vi "Register gRPC Methods.vi"(8 "error in (no error)":errorcluster, 11 "Template Server in":refnum<class "TestService.lvclass">) -> (0 "error out":errorcluster, 3 "Template Server out":refnum<class "TestService.lvclass">)   [LabVIEW 2021, in "test_service_server.lvlib" / "TestService.lvclass"]
uses:
  TestService.lvclass
  typeDefs/Server Internal UEs.ctl
  typeDefs/Server Internal Message.ctl
  typeDefs/Server gRPC UEs.ctl
  <vilib>/gRPC/LabVIEW gRPC Library/Server API/typeDefs/gRPCId Cluster.ctl
  <vilib>/gRPC/LabVIEW gRPC Library/Shared/grpcId.ctl
  TestService.lvclass/TestService.ctl
  <vilib>/gRPC/LabVIEW gRPC Library/grpc-lvsupport-release.lvlib
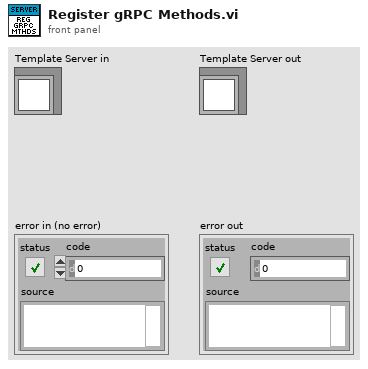
[diagram p1: front panel]
types:
  T1 = typedef "test_service_server.lvlib/TestService.lvclass/Server gRPC UEs.ctl" = cluster{"TestService Method1 gRPC UE":refnum<user-event>, "TestService Method2 gRPC UE":refnum<user-event>, "TestService Method3 gRPC UE":refnum<user-event>, "TestService Method4 gRPC UE":refnum<user-event>}
  T2 = typedef "test_service_server.lvlib/TestService.lvclass/Server Internal UEs.ctl" = cluster{"TestService Method1 Internal UE":refnum<user-event>, "TestService Method2 Internal UE":refnum<user-event>, "TestService Method3 Internal UE":refnum<user-event>, "TestService Method4 Internal UE":refnum<user-event>}
  T3 = typedef "grpc-lvsupport-release.lvlib/grpcId.ctl" = u64
  T4 = typedef "test_service_server.lvlib/TestService.lvclass/Server Internal Message UE.ctl" = refnum<user-event>
  T5 = typedef "grpc-lvsupport-release.lvlib/gRPCId Cluster UE.ctl" = refnum<user-event>
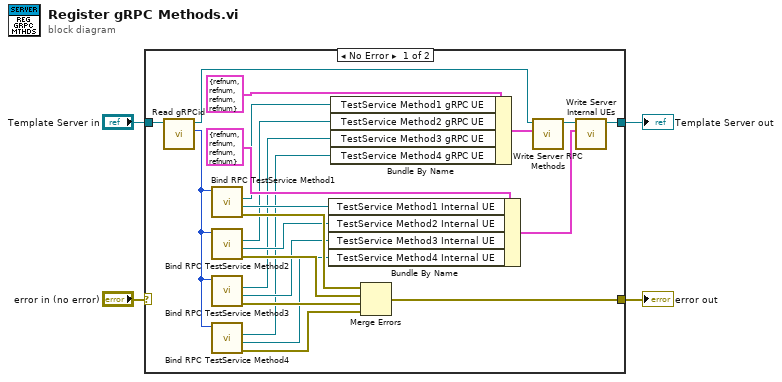
[diagram p0: block diagram]
diagram:
  n1 = case shown="No Error" "error in (no error)" {
    selector: "error in (no error)" -> [_ w27]
    tunnel: "Template Server in" -> [w18 w28]
    tunnel: [w26 w27] -> w3
    tunnel: [w25 w28] -> w2
    frame No Error {
      n2 = call-dynamic "Read gRPCid.vi"("iService in"=w18) -> ("gRPCid"=w17:T3, "iService out"=w19:refnum<class "TestService.lvclass">)  [unwired: 8 in, 1 out]
      n3 = call "Bind RPC TestService Method1.vi"("gRPCid server in"=w17) -> ("error out"=w16:errorcluster, "TestService Method1 Internal UE"=w14:T4, "TestService Method1 gRPC UE"=w15:T5)  [unwired: 7 in, 1 out]
      n4 = call "Bind RPC TestService Method2.vi"("gRPCid server in"=w17) -> ("error out"=w13:errorcluster, "TestService Method2 Internal UE"=w11:T4, "TestService Method2 gRPC UE"=w12:T5)  [unwired: 7 in, 1 out]
      n5 = call "Bind RPC TestService Method3.vi"("gRPCid server in"=w17) -> ("error out"=w10:errorcluster, "TestService Method3 Internal UE"=w8:T4, "TestService Method3 gRPC UE"=w9:T5)  [unwired: 7 in, 1 out]
      n6 = call "Bind RPC TestService Method4.vi"("gRPCid server in"=w17) -> ("error out"=w7:errorcluster, "TestService Method4 Internal UE"=w5:T4, "TestService Method4 gRPC UE"=w6:T5)  [unwired: 7 in, 1 out]
      n7 = Bundle By Name ("Bundle Internal UEs")(cluster=T2 {"TestService Method1 Internal UE"=refnum, "TestService Method2 Internal UE"=refnum, "TestService Method3 Internal UE"=refnum, "TestService Method4 Internal UE"=refnum} ("Server Internal UEs"), "TestService Method1 Internal UE"=w14, "TestService Method2 Internal UE"=w11, "TestService Method3 Internal UE"=w8, "TestService Method4 Internal UE"=w5) -> (w24:T2)
      n8 = Bundle By Name ("Bundle gRPC UEs")(cluster=T1 {"TestService Method1 gRPC UE"=refnum, "TestService Method2 gRPC UE"=refnum, "TestService Method3 gRPC UE"=refnum, "TestService Method4 gRPC UE"=refnum} ("gRPC Server Method Events"), "TestService Method1 gRPC UE"=w15, "TestService Method2 gRPC UE"=w12, "TestService Method3 gRPC UE"=w9, "TestService Method4 gRPC UE"=w6) -> (w21:T1)
      n9 = Merge Errors(w16, w13, w10, w7) -> (w26:errorcluster)
      n10 = call "Write Server RPC Methods.vi"("Server RPC Methods"=w21, "SignalGeneratorService in"=w19) -> ("SignalGeneratorService out"=w22:refnum<class "TestService.lvclass">)  [unwired: 8 in, 1 out]
      n11 = call "Write Server Internal UEs.vi"("Server Internal UEs"=w24, "SignalGeneratorService in"=w22) -> ("SignalGeneratorService out"=w25:refnum<class "TestService.lvclass">)  [unwired: 8 in, 1 out]
    }
    frame Error {
    }
  }
  "error out" <- w3
  "Template Server out" <- w2
